vi "Thumbstick Config.vi"(0 "Arduino Resource":T1={"COM Port"="", "Board Type"=enum."ChipKit uC32", "Connection Type"=enum."USB / Serial", "Baud Rate (115200)"=15, "Bytes Per Packet (15)"=15}, 5 "Horizontal Axis AI Pin":u8, 7 "Vertical Axis AI Pin":u8, 9 "Select DI Pin":u8, 11 "error in":errorcluster) -> (4 "Arduino Resource":T1={"COM Port"="", "Board Type"=enum."ChipKit uC32", "Connection Type"=enum."USB / Serial", "Baud Rate (115200)"=15, "Bytes Per Packet (15)"=15}, 8 "Thumbstick Data":T4, 15 "error out":errorcluster)   [LabVIEW 2011, in "LabVIEW Interface for ChipKit.lvlib"]
doc: "Configure two Arduino analog inputs and one Arduino digital input for use with a thumb stick."
uses:
  LabVIEW Interface for ChipKit.lvlib
  Private/Type Defs/Pin Mode.ctl
  Private/Type Defs/Board Type.ctl
  Private/Type Defs/Chipkit Resource.ctl
  Private/Type Defs/Connection Type.ctl
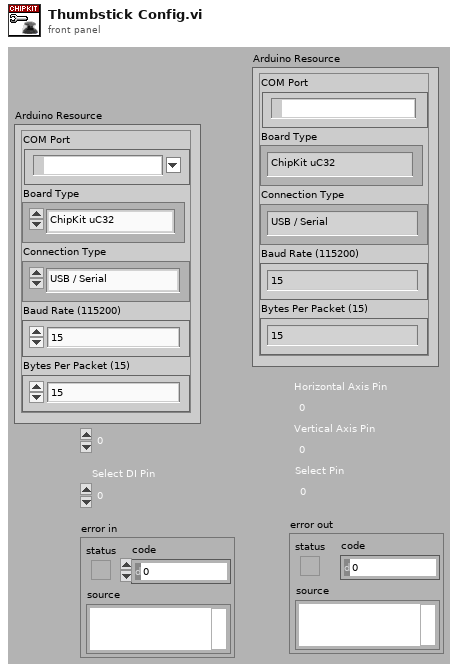
[diagram p1: front panel]
types:
  T1 = typedef "LabVIEW Interface for ChipKit.lvlib/Chipkit Resource.ctl" = cluster{"COM Port":refnum<visa-resource-name>, "Board Type":T2, "Connection Type":T3, "Baud Rate (115200)":u32, "Bytes Per Packet (15)":u32}
  T2 = typedef "LabVIEW Interface for ChipKit.lvlib/Board Type.ctl" = enum16{"ChipKit uC32", "ChipKit Uno32", "ChipKit Max32"}
  T3 = typedef "LabVIEW Interface for ChipKit.lvlib/Connection Type.ctl" = enum8{"USB / Serial", "XBEE", "BlueSmirf (Bluetooth)"}
  T4 = cluster{"Horizontal Axis Pin":dbl, "Vertical Axis Pin":dbl, "Select Pin":dbl}
  T5 = typedef "LabVIEW Interface for ChipKit.lvlib/Pin Mode.ctl" = enum8{"Input", "Output"}
  T6 = cluster{"Horizontal Axis AI Pin":u8, "Vertical Axis AI Pin":u8, "Select DI Pin":u8}
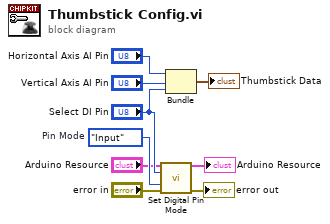
[diagram p0: block diagram]
diagram:
  w7 = Pin_Mode."Input"  # Pin Mode
  n1 = call "Set Digital Pin Mode.vi"("Arduino Resource"="Arduino Resource", "Digital I/O Pin"="Select DI Pin", "Pin Mode (Input)"=w7, "error in"="error in") -> ("Arduino Resource"=→"Arduino Resource":T1, "error out"=→"error out":errorcluster)  [unwired: 10 in]
  n2 = Bundle("Horizontal Axis AI Pin"="Horizontal Axis AI Pin", "Vertical Axis AI Pin"="Vertical Axis AI Pin", "Select DI Pin"="Select DI Pin") -> (→"Thumbstick Data":T6)  [unwired: 1 in]
